vi "CS POLARIS BME DG.CheckIn DG_System.vi"(7 "error in":errorcluster, 8 "timeout in ms (-1)":i32, 9 "BME_DG_System":refnum<class "BME_DG_System.lvclass">, 10 "i ref in":refnum<vi>) -> (0 "error in":errorcluster, 3 "i ref out":refnum<vi>)   [LabVIEW 2009, in "CS POLARIS BME DG.lvlib"]
uses:
  CS POLARIS BME DG.lvlib
  DG Classes/BME_DG_System/BME_DG_System.lvclass
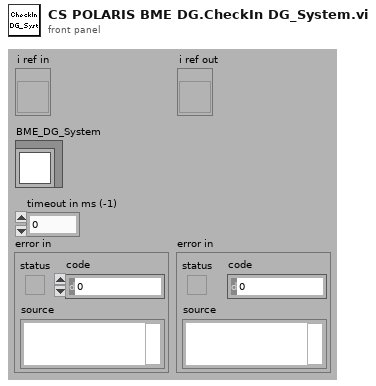
[diagram p1: front panel]
types:
  T1 = typedef "CS POLARIS BME DG.lvlib/CS POLARIS BME DG.i attribute.ctl" = cluster{"Numeric":dbl, "DG_System":refnum<queue>, "UpdateTasks":refnum<queue>}
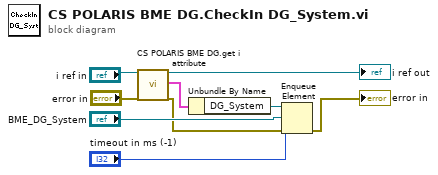
[diagram p0: block diagram]
diagram:
  n1 = call "CS POLARIS BME DG.get i attribute.vi"("i ref in"="i ref in", "error in (no error)"="error in") -> ("i ref out"=→"i ref out":refnum<vi>, "i attribute"=w3:T1, "error out"=w4:errorcluster)  [unwired: 15 in]
  n2 = Unbundle By Name(w3) -> ("DG_System"=w2:refnum<queue>)
  n3 = Enqueue Element(queue=w2, element="BME_DG_System", timeout in ms (-1)="timeout in ms (-1)", error in (no error)=w4) -> (error out=→"error in":errorcluster)  [unwired: 2 out]
